vi "format_progressbar.vi"(3 "# itx files":i32) -> (1 "progbar msg":string)   [LabVIEW 2016]
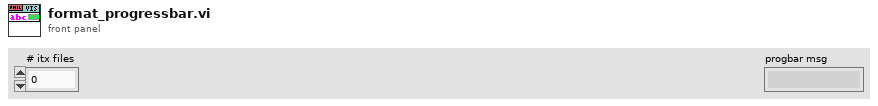
[diagram p1: front panel]
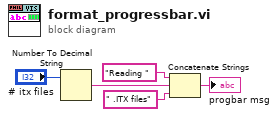
[diagram p0: block diagram]
diagram:
  n1 = Number To Decimal String(number="# itx files") -> (decimal integer string=w5:string)  [unwired: 1 in]
  n2 = Concatenate Strings("Reading " ("title (\"Progress\")"), w5, " .ITX files" ("title (\"Progress\")")) -> (→"progbar msg":string)
